vi "Diagnostic Logger v1.7.vi"() -> ()   [LabVIEW 2014]
uses:
  <vilib>/Rock Robotics/WPI/DriverStation/WPI_DriverStationRobotMode2.ctl
  <vilib>/Utility/file.llb/Write To Spreadsheet File (DBL).vi
  Begin/Global Variables.vi
panel:
  out "nRef":refnum<notifier>
  # "CSV Columns Transposed:\n\n01 - Robot Mode (0=?, 1=Auton, 2=Teleop)\n02 - Elapsed Time (ms)\n03 - dt (ms)\n04 - Gyro Yaw\n05 - Gyro Pitch\n06 - Gyro Roll\n07 - Driver JS LX\n08 - Driver JS LY\n09 - Driver JS RX\n10 - Drive Resolver FL\n11 - Drive Resolver FR\n12 - Drive Resolver BL\n13 - Drive Resolver BR\n14 - Drive Encoder FL\n15 - Drive Encoder FR\n16 - Drive Encoder BL\n17 - Drive Encoder BR\n18 - Drive Speed FL\n19 - Drive Speed FR\n20 - Drive Speed BL\n21 - Drive Speed BR\n22 - Lift Height Left\n23 - Lift Height Right\n24 - Lift Rate Left\n25 - Lift Rate Right"
  # "Data Usage Rates:\n\n20 KB / sec\n1.2 MB / min\n72 MB / hour"
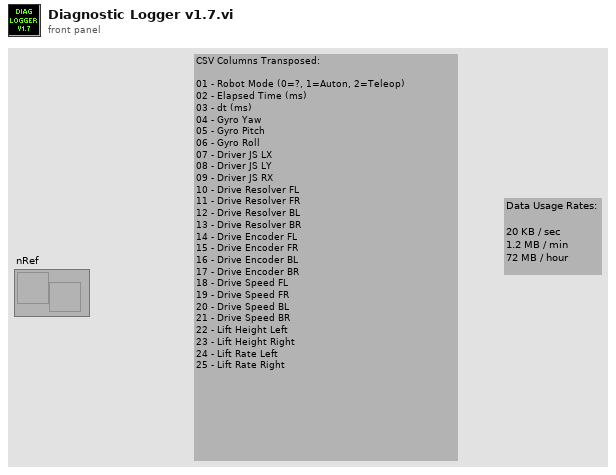
[diagram p1: front panel]
types:
  T1 = typedef "WPI_DriverStationRobotMode2.ctl" = enum16{"Autonomous Disabled", "Autonomous Enabled", "Teleop Disabled", "Teleop Enabled", "Disconnected", "Finish", "Test Disabled", "Test Enabled", "Emergency Stopped"}
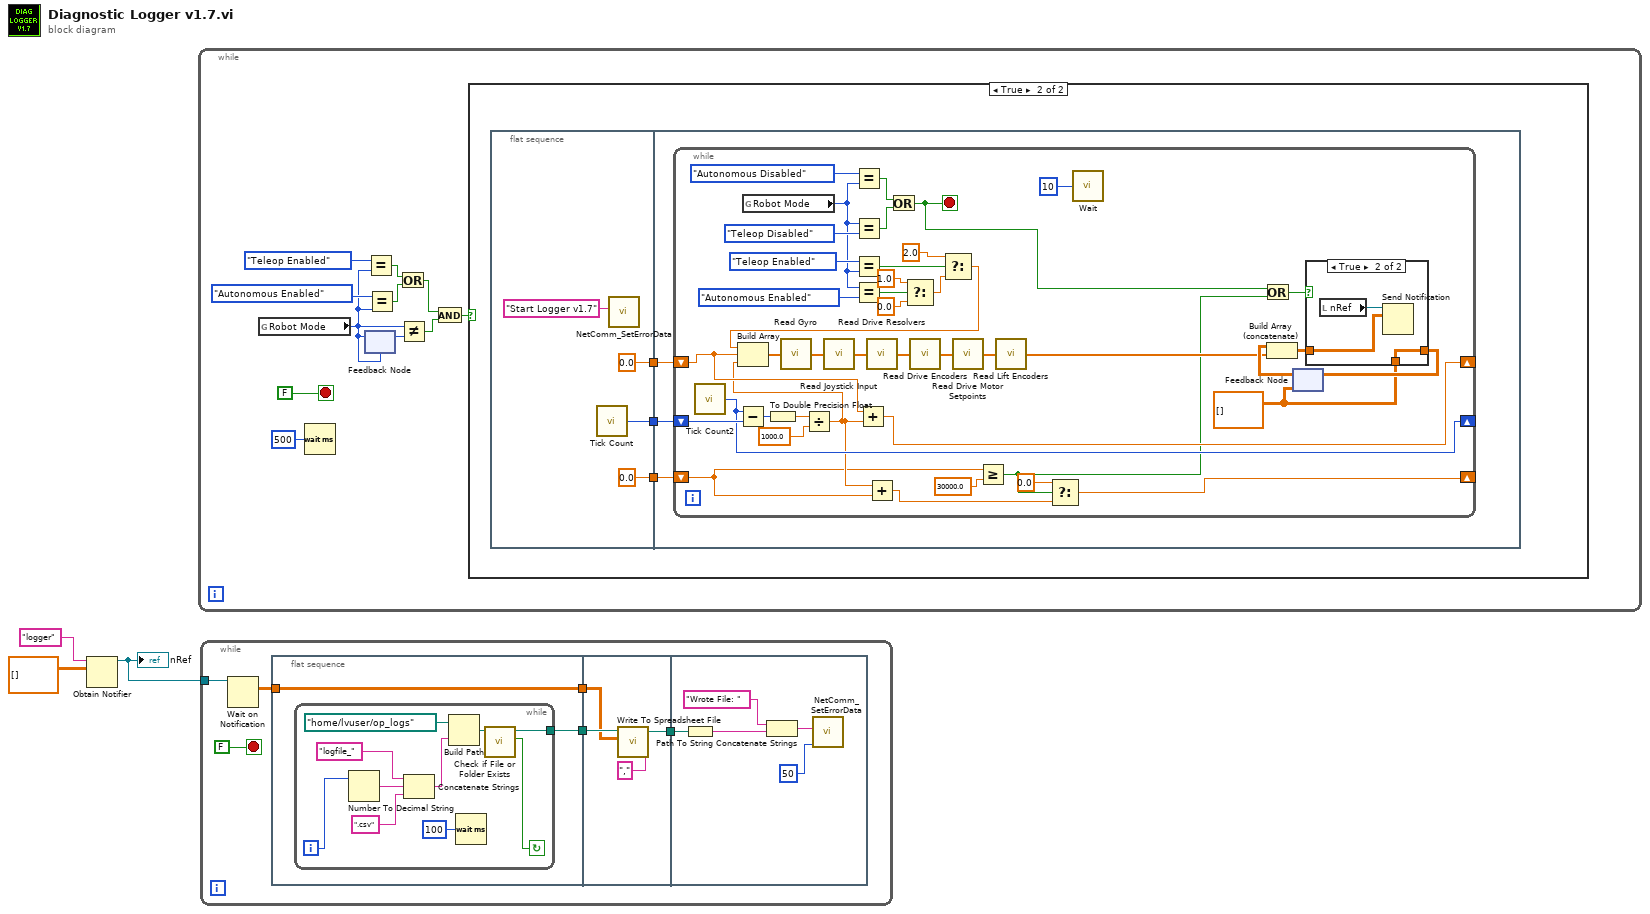
[diagram p0: block diagram]
diagram:
  n1 = Obtain Notifier(name (unnamed)="logger", notification data type=dbl[][] []) -> (notifier out=w1:refnum<notifier>)  [unwired: 2 in, 2 out]
  "nRef" <- w1
  n2 = while {
    stop <- FALSE stop-if-true
    n3 = global read "Global Variables.vi" "Robot Mode"() -> (w9:T1)
    n4 = Wait (ms)(milliseconds to wait=u32 500) -> ()  [unwired: 1 out]
    n5 = feedback-in #1(w9) -> ()
    n6 = feedback #1(w9) -> (w13:T1)
    n7 = Equal?(x=WPI_DriverStationRobotMode2."Teleop Enabled", y=w9) -> (x = y?=w8:bool)
    n8 = Equal?(x=WPI_DriverStationRobotMode2."Autonomous Enabled", y=w9) -> (x = y?=w7:bool)
    n9 = Or(x=w8, y=w7) -> (x .or. y?=w6:bool)
    n10 = Not Equal?(x=w9, y=w13) -> (x != y?=w12:bool)
    n11 = And(x=w6, y=w12) -> (x .and. y?=w5:bool)
    n12 = case shown="True" w5 {
      frame False {
      }
      frame True {
        n13 = flat-sequence {
          tunnel: [w20] -> w17
          tunnel: [0.0] -> w16
          tunnel: [0.0] -> w15
          tunnel: w17 -> [w24]
          tunnel: w16 -> [w23]
          tunnel: w15 -> [w22]
          frame #0 {
            n14 = call "Tick Count"() -> ("Tick Count(uSec)"=w20:u32)
            n15 = call <vilib>:"NetComm_SetErrorData.vi"("Error Data"="Start Logger v1.7") -> ()  [unwired: 3 in, 8 out]
          }
          frame #1 {
            n16 = while {
              shift-right: [w37] -> _
              shift-left: w24 -> [w38]
              shift-right: [w33] -> _
              shift-left: w23 -> [w31]
              shift-right: [w28] -> _
              shift-left: w22 -> [w26]
              stop <- w39 stop-if-true
              w42 = dbl[][] []
              n17 = call "Tick Count2"() -> ("Tick Count(uSec)"=w37:u32)
              n18 = Subtract(x=w37, y=w38) -> (x-y=w36:u32)
              n19 = global read "Global Variables.vi" "Robot Mode"() -> (w59:T1)
              n20 = To Double Precision Float(number=w36) -> (double precision float=w35:dbl)
              n21 = Divide(x=w35, y=1000.0) -> (x/y=w27:dbl)
              n22 = Equal?(x=WPI_DriverStationRobotMode2."Autonomous Disabled", y=w59) -> (x = y?=w63:bool)
              n23 = Equal?(x=w59, y=WPI_DriverStationRobotMode2."Teleop Disabled" ("x")) -> (x = y?=w64:bool)
              n24 = Equal?(x=WPI_DriverStationRobotMode2."Teleop Enabled", y=w59) -> (x = y?=w61:bool)
              n25 = Equal?(x=w59, y=WPI_DriverStationRobotMode2."Autonomous Enabled" ("x")) -> (x = y?=w58:bool)
              n26 = Add(x=w31, y=w27) -> (x+y=w33:dbl)
              n27 = Add(x=w27, y=w26) -> (x+y=w25:dbl)
              n28 = Or(x=w63, y=w64) -> (x .or. y?=w39:bool)
              n29 = Select(t=1.0, s=w58, f=0.0) -> (s? t:f=w57:dbl)
              n30 = Select(t=2.0, s=w61, f=w57) -> (s? t:f=w46:dbl)
              n31 = Build Array(w46, w31, w27) -> (w47:dbl[])
              n32 = call "Read Gyro.vi"("Input Array"=w47) -> ("Appended Array"=w52:dbl[])
              n33 = call "Read Joystick Input.vi"("Input Array"=w52) -> ("Appended Array"=w51:dbl[])
              n34 = call "Read Drive Resolvers.vi"("Input Array"=w51) -> ("Appended Array"=w50:dbl[])
              n35 = call "Read Drive Encoders.vi"("Input Array"=w50) -> ("Appended Array"=w49:dbl[])  [unwired: 10 in, 4 out]
              n36 = call "Read Drive Motor Setpoints.vi"("Input Array"=w49) -> ("Appended Array"=w48:dbl[])
              n37 = Greater Or Equal?(x=w26, y=30000.0) -> (x >= y?=w30:bool)
              n38 = call "Read Lift Encoders.vi"("Input Array"=w48) -> ("Appended Array"=w45:dbl[])
              n39 = Select(t=0.0, s=w30, f=w25) -> (s? t:f=w28:dbl)
              n40 = call "Wait"("Count(mSec)"=u32 10) -> ()  [unwired: 1 out]
              n41 = Or(x=w39, y=w30) -> (x .or. y?=w40:bool)
              n42 = feedback #2(w42) -> (w53:dbl[][])
              n43 = Build Array (concatenate)(w53, w45) -> (w44:dbl[][])
              n44 = case shown="True" w40 {
                tunnel: w44 -> [w67 w69]
                tunnel: [w67 w70] -> w43
                tunnel: w42 -> [_ w70]
                frame False {
                }
                frame True {
                  n45 = local read "nRef"() -> (w68:refnum<notifier>)
                  n46 = Send Notification(notification=w69, notifier=w68) -> ()  [unwired: 1 in, 2 out]
                }
              }
              n47 = feedback-in #2(w43) -> ()
            }
          }
        }
      }
    }
  }
  n48 = while {
    tunnel: w1 -> [w71]
    stop <- FALSE stop-if-true
    n49 = Wait on Notification(notifier=w71) -> (notification=w75:dbl[][])  [unwired: 3 in, 3 out]
    n50 = flat-sequence {
      tunnel: w75 -> [w78]
      tunnel: [w78] -> w74
      tunnel: [w77] -> w73
      tunnel: w74 -> [w90]
      tunnel: w73 -> [w91]
      tunnel: [w89] -> w72
      tunnel: w72 -> [w93]
      frame #0 {
        n51 = while {
          tunnel: [w81] -> w77
          i -> [w80]
          stop <- w88 continue-if-true
          n52 = Number To Decimal String(number=w80) -> (decimal integer string=w85:string)  [unwired: 1 in]
          n53 = Concatenate Strings("logfile_", w85, ".csv") -> (w84:string)
          n54 = Build Path(base path=path "/home/lvuser/op_logs" ("file path (dialog if empty)"), name or relative path=w84) -> (appended path=w87:path)
          n55 = Wait (ms)(milliseconds to wait=u32 100) -> ()  [unwired: 1 out]
          n56 = call <vilib>:"Check if File or Folder Exists.vi"("path"=w87) -> ("file or folder exists?"=w88:bool, "dup path"=w81:path)  [unwired: 8 in, 1 out]
        }
      }
      frame #1 {
        n57 = call-poly <vilib>:"Write To Spreadsheet File.vi"("delimiter (\\t)"="," ("delimiter (\\t)"), "2D data"=w90, "file path (dialog if empty)"=w91) -> ("new file path (Not A Path if cancelled)"=w89:path)  [unwired: 5 in]
      }
      frame #2 {
        n58 = Path To String(path=w93) -> (string=w94:string)
        n59 = Concatenate Strings("Wrote File: ", w94) -> (w96:string)
        n60 = call <vilib>:"NetComm_SetErrorData.vi"("Timeout (ms)"=50, "Error Data"=w96) -> ()  [unwired: 2 in, 8 out]
      }
    }
  }
